vi "导入Excel.vi"(8 "error in (no error)":errorcluster) -> (0 "error out":errorcluster, 3 "data":string[][](array[string]))   [LabVIEW 2016, in "Alarm interface.lvlib"]
uses:
  Alarm interface.lvlib
  <vilib>/addons/_office/excel.llb/Excel Get Data ([str]).vi
  <vilib>/regexp/Match Regular Expression.xnode
  <vilib>/Utility/NIReport.llb/NI_report.lvclass
  <vilib>/Utility/NIReport.llb/Excel/NI_Excel.lvclass
  <vilib>/addons/_office/NI_ReportGenerationToolkit.lvlib
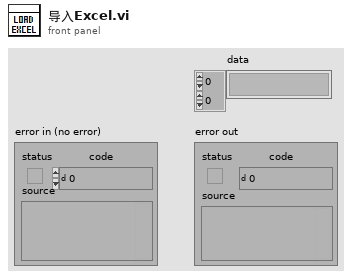
[diagram p1: front panel]
types:
  T1 = enum16{"Standard Report", "HTML", "Word", "Excel"}
  T2 = enum16{"maximized", "minimized", "normal", "no change"}
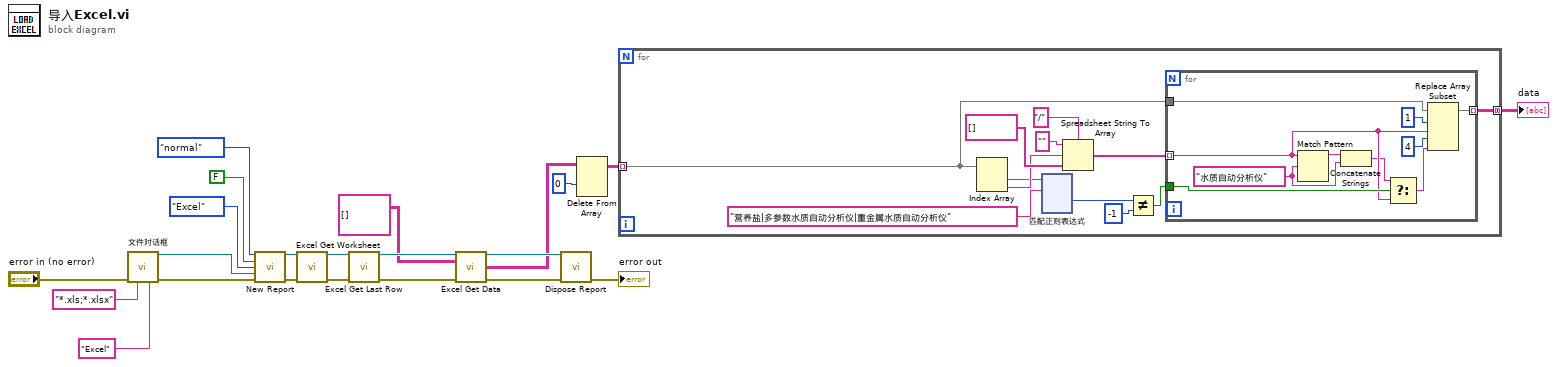
[diagram p0: block diagram]
diagram:
  n1 = call "文件对话框"("error in"="error in (no error)", "pattern (all files)"="*.xls;*.xlsx" ("pattern label"), "pattern label"="Excel" ("pattern (all files)")) -> ("selected path"=w10:path, "error out"=w9:errorcluster)  [unwired: 9 in, 2 out]
  n2 = call <vilib>:"New Report.vi"("window state (normal)"=T2."normal", "display alerts? (F)"=FALSE, "report type"=T1."Excel", "template (empty)"=w10, "error in (no error)"=w9) -> ("report out"=w17:refnum<class "NI_report.lvclass">, "error out"=w11:errorcluster)  [unwired: 9 in]
  n3 = call <vilib>:"Excel Get Worksheet.vi"("report in"=w17, "error in (no error)"=w11) -> ("report out"=w22:refnum<class "NI_report.lvclass">, "error out"=w21:errorcluster)  [unwired: 12 in]
  n4 = call <vilib>:"Excel Get Last Row.vi"("report in"=w22, "error in (no error)"=w21) -> ("report out"=w20:refnum<class "NI_report.lvclass">, "error out"=w19:errorcluster)  [unwired: 11 in, 1 out]
  n5 = call-poly <vilib>:"Excel Get Data.vi"("report in"=w20, "data type"=string[][] [], "error in (no error)"=w19) -> ("report out"=w16:refnum<class "NI_report.lvclass">, "data"=w5:string[][], "error out"=w15:errorcluster)  [unwired: 10 in]
  n6 = call-dynamic "Dispose Report.vi"("report in"=w16, "error in (no error)"=w15) -> ("error out"=→"error out":errorcluster)  [unwired: 13 in]
  n7 = Delete From Array(array=w5, index (row)=0 ("索引 (行)")) -> (array with subset deleted=w6:string[][])  [unwired: 2 in, 1 out]
  n8 = for {
    tunnel: w6 -> [w30] mode=indexing
    tunnel: [w29] -> w1 mode=concatenating
    n9 = Index Array(array=w30) -> (element #1=w23:string, element #2=w24:string)  [unwired: 2 in]
    n10 = xnode "匹配正则表达式"("输入字符串"=w23, "正则表达式"="营养盐|多参数水质自动分析仪|重金属水质自动分析仪") -> ("匹配后偏移量"=w25:i32)  [unwired: 4 in, 4 out]
    n11 = Spreadsheet String To Array(delimiter (Tab)="/" ("分隔符(Tab)"), format string="" ("格式字符串"), spreadsheet string=w24, array type (2D Dbl)=string[] []) -> (array=w31:string[])
    n12 = Not Equal?(x=w25, y=-1) -> (x != y?=w26:bool)
    n13 = for {
      tunnel: w31 -> [w152] mode=indexing
      tunnel: w30 -> [w158]
      tunnel: [w155] -> w29 mode=indexing
      tunnel: w26 -> [w154]
      w150 = "水质自动分析仪" ("正则表达式")
      n14 = Match Pattern(string=w152, regular expression=w150) -> (before substring=w151:string)  [unwired: 1 in, 3 out]
      n15 = Concatenate Strings(w151, w150) -> (w149:string)
      n16 = Select(t=w149, s=w154, f=w152) -> (s? t:f=w153:string)
      n17 = Replace Array Subset(array=w158, new element #1=w152, index #1=1 ("索引"), new element #2=w153, index #2=4 ("索引")) -> (w155:string[])
    }
  }
  "data" <- w1
